vi "TCP-MyCLient.vi"() -> ()   [LabVIEW 2020]
panel:
  out "number":i32
  out "Waveform Chart":i32(graph)
  out "error out":errorcluster
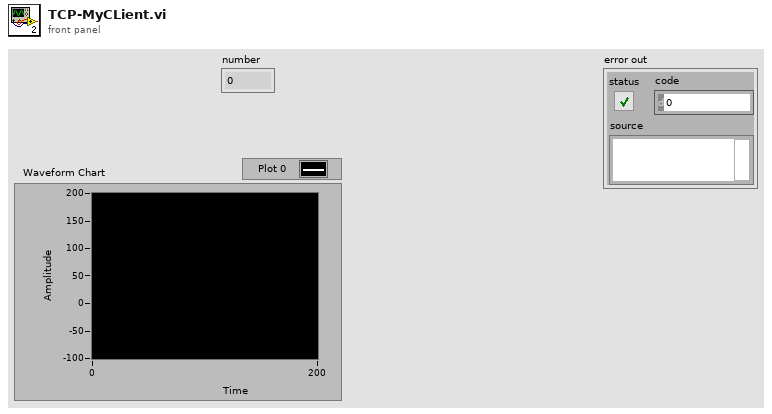
[diagram p1: front panel]
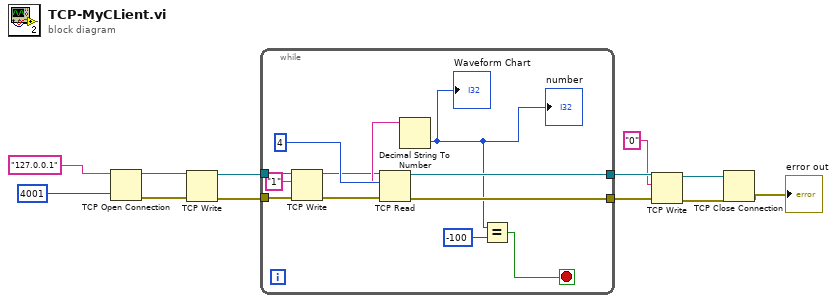
[diagram p0: block diagram]
diagram:
  n1 = TCP Open Connection(address="127.0.0.1", remote port or service name=u16 4001) -> (connection ID=w6:refnum<k5>, error out=w7:errorcluster)  [unwired: 3 in]
  n2 = TCP Write(connection ID=w6, error in (no error)=w7) -> (connection ID out=w9:refnum<k5>, error out=w8:errorcluster)  [unwired: 2 in, 1 out]
  n3 = while {
    tunnel: w9 -> [w20]
    tunnel: w8 -> [w21]
    tunnel: [w16] -> w3
    tunnel: [w24] -> w2
    stop <- w15 stop-if-true
    n4 = TCP Write(connection ID=w20, data in="1", error in (no error)=w21) -> (connection ID out=w19:refnum<k5>, error out=w18:errorcluster)  [unwired: 1 in, 1 out]
    n5 = TCP Read(connection ID=w19, bytes to read=4, error in (no error)=w18) -> (connection ID out=w16:refnum<k5>, data out=w22:string, error out=w24:errorcluster)  [unwired: 2 in]
    n6 = Decimal String To Number(string=w22) -> (number=w14:i32)  [unwired: 2 in, 1 out]
    "number" <- w14
    "Waveform Chart" <- w14
    n7 = Equal?(x=w14, y=-100) -> (x = y?=w15:bool)
  }
  n8 = TCP Write(connection ID=w3, data in="0", error in (no error)=w2) -> (connection ID out=w4:refnum<k5>, error out=w5:errorcluster)  [unwired: 1 in, 1 out]
  n9 = TCP Close Connection(connection ID=w4, error in (no error)=w5) -> (error out=→"error out":errorcluster)  [unwired: 1 in, 1 out]
